vi "Get Loop Period (us).vi"() -> (3 "Loop Period (us)":u32)   [LabVIEW 2017]
doc: "Returns loop period in units of us."
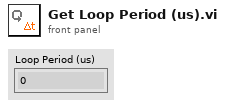
[diagram p1: front panel]
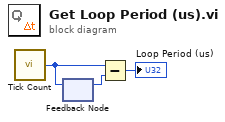
[diagram p0: block diagram]
diagram:
  n1 = call "Tick Count"() -> ("Tick Count(uSec)"=w3:u32)
  n2 = feedback #1() -> (w2:u32)  [unwired: 1 in]
  n3 = feedback-in #1(w3) -> ()
  n4 = Subtract(x=w3, y=w2) -> (x-y=→"Loop Period (us)":u32)
